vi "Angle to hub.vi"(2 "Robot Velocities In":T1={"X Velocity"=0.0, "Y Velocity"=-0.0, "Rotational \nVelocity"=0.0}, 3 "Time in flight":dbl) -> (0 "Distance to hub":dbl, 1 "Angle to hub":dbl)   [LabVIEW 2025]
uses:
  Rebuilt-Apprentice/swerve-template/Type Definitions/Data/Robot Velocities.ctl
  <vilib>/Rock Robotics/WPI/DriverStation/WPI_DriverStationAllianceInfo.ctl
  <vilib>/Rock Robotics/Network Tables/NT Read Numeric Array.vi
panel:
  # "distance off the hub"
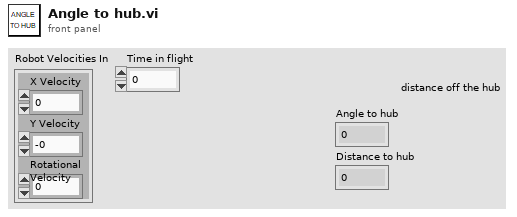
[diagram p1: front panel]
types:
  T1 = typedef "Robot Velocities.ctl" = cluster{"X Velocity":dbl, "Y Velocity":dbl, "Rotational \nVelocity":dbl}
  T2 = typedef "WPI_DriverStationAllianceInfo.ctl" = enum16{"Red", "Blue", "Invalid"}
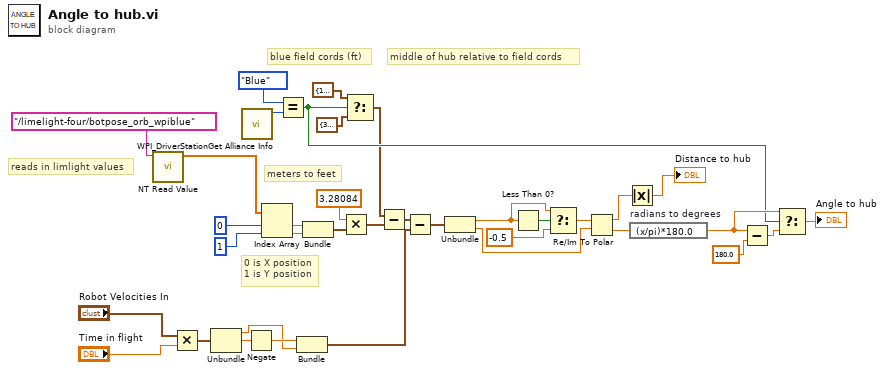
[diagram p0: block diagram]
diagram:
  # "blue field cords (ft)"
  # "middle of hub relative to field cords"
  # "meters to feet"
  # "reads in limlight values"
  # "0 is X position\n1 is Y position"
  n1 = call-poly <vilib>:"NT Read Value.vi"("name"="/limelight-four/botpose_orb_wpiblue") -> ("value"=w21:dbl[])  [unwired: 8 in, 2 out]
  n2 = Multiply(x="Robot Velocities In", y="Time in flight") -> (x*y=w15:T1)
  n3 = Unbundle(w15) -> ("X Velocity"=w9:dbl, "Y Velocity"=w10:dbl)  [unwired: 1 out]
  n4 = call <vilib>:"WPI_DriverStationGet Alliance Info.vi"() -> ("Alliance"=w28:T2)  [unwired: 6 in, 5 out]
  n5 = Negate(x=w10) -> (-x=w14:dbl)
  n6 = Index Array(array=w21, index #1=0 ("index"), index #2=1 ("index")) -> (element #1=w23:dbl, element #2=w24:dbl)
  n7 = Equal?(x=WPI_DriverStationAllianceInfo."Blue", y=w28) -> (x = y?=w30:bool)
  n8 = Bundle(w14, "X Velocity"=w9) -> (w11:cluster{dbl, "X Velocity":dbl})  [unwired: 1 in]
  n9 = Bundle("Numeric"=w23, "Numeric"=w24) -> (w22:cluster{"Numeric":dbl, "Numeric":dbl})  [unwired: 1 in]
  n10 = Multiply(x=3.28084, y=w22) -> (x*y=w25:cluster{"Numeric":dbl, "Numeric":dbl})
  n11 = Select(t=cluster{"Numeric":dbl, "Numeric":dbl} {"Numeric"=15.31, "Numeric"=13.19333} ("x"), s=w30, f=cluster{"Numeric":dbl, "Numeric":dbl} {"Numeric"=39.04667, "Numeric"=13.19333} ("x")) -> (s? t:f=w13:cluster{"Numeric":dbl, "Numeric":dbl})
  n12 = Subtract(x=w13, y=w25) -> (x-y=w12:cluster{"Numeric":dbl, "Numeric":dbl})
  n13 = Subtract(x=w12, y=w11) -> (x-y=w7:cluster{dbl, dbl})
  n14 = Unbundle(w7) -> (w6:dbl, w3:dbl)
  n15 = Less Than 0?(x=w6) -> (x < 0?=w8:bool)
  n16 = Select(t=w6, s=w8, f=-0.5 ("t")) -> (s? t:f=w5:dbl)
  n17 = Re/Im To Polar(2:w3, 3:w5) -> (0:w31:dbl, 1:w33:dbl)
  n18 = Absolute Value(x=w33) -> (abs(x)=→"Distance to hub":dbl)
  n19 = expression code="(x/pi)*180.0" "radians to degrees"(w31) -> (w35:dbl)
  n20 = Subtract(x=w35, y=180.0 ("x")) -> (x-y=w32:dbl)
  n21 = Select(t=w35, s=w30, f=w32) -> (s? t:f=→"Angle to hub":dbl)
